vi "Unflatten Waveform Summary JSON.vi"(8 "error in":errorcluster, 11 "Measurement Configuration In":T1={"TDMS File Location"="", "Run Action"="Create/Replace Wfm Group", "Wfm Group Name"="Wfm1", "Channel Names"=[], "Waveforms Summary JSON"=[]}) -> (0 "error out":errorcluster, 2 "Waveforms":waveform(dbl)[](array[waveform]), 3 "Measurement Configuration Out":T1)   [LabVIEW 2025, in "TDMS Waveform Creator.lvclass"]
uses:
  TDMS Waveform Creator.lvclass
  TDMS Waveform Creator.lvclass/TDMS Waveform Creator.ctl
  TDMS Waveform Creator UI/TDMS Waveform Creator UI.lvlib
  Measurement Configuration.ctl
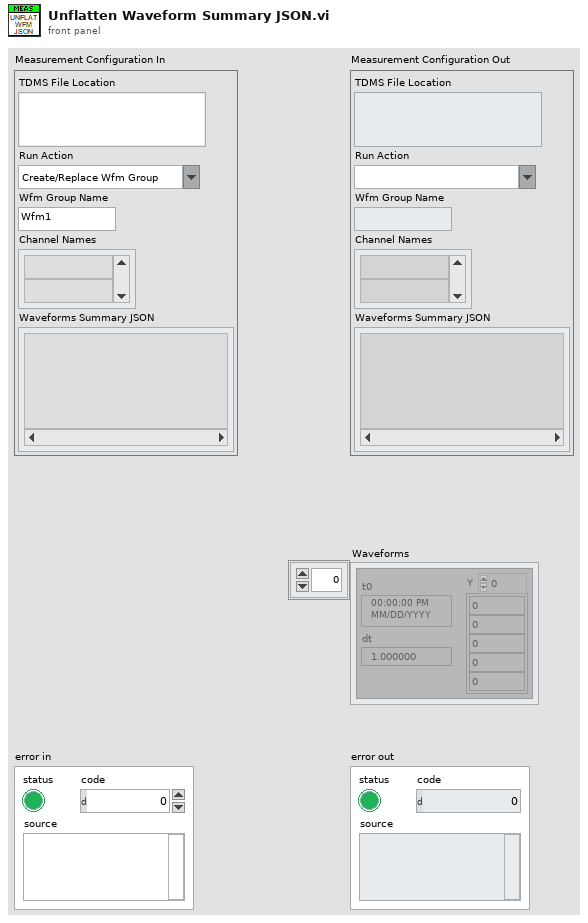
[diagram p1: front panel]
types:
  T1 = typedef "TDMS Waveform Creator.lvclass/Measurement Configuration.ctl" = cluster{"TDMS File Location":string, "Run Action":string, "Wfm Group Name":string, "Channel Names":string[], "Waveforms Summary JSON":string[]}
  T2 = cluster{"Trim and Resample Settings":cluster{"Duration":dbl, "Sample Rate":dbl}, "Wfms Json":string[]}
  T3 = cluster{"File Path":string, "Sample Rate (Hz)":dbl, "Read From":i32, "Pre Delay (s)":dbl, "Post Delay (s)":dbl, "Scale":dbl}
  T4 = cluster{"Waveform Type":i32, "Sample Rate (Hz)":dbl, "Frequency (Hz)":dbl, "Amplitude":dbl, "Number of Cycles":u32, "Ramp Start":dbl, "Ramp Stop":dbl, "Length (s)":dbl, "DC Value":dbl, "Duration (s)":dbl, "Pre Delay (s)":dbl, "Post Delay (s)":dbl}
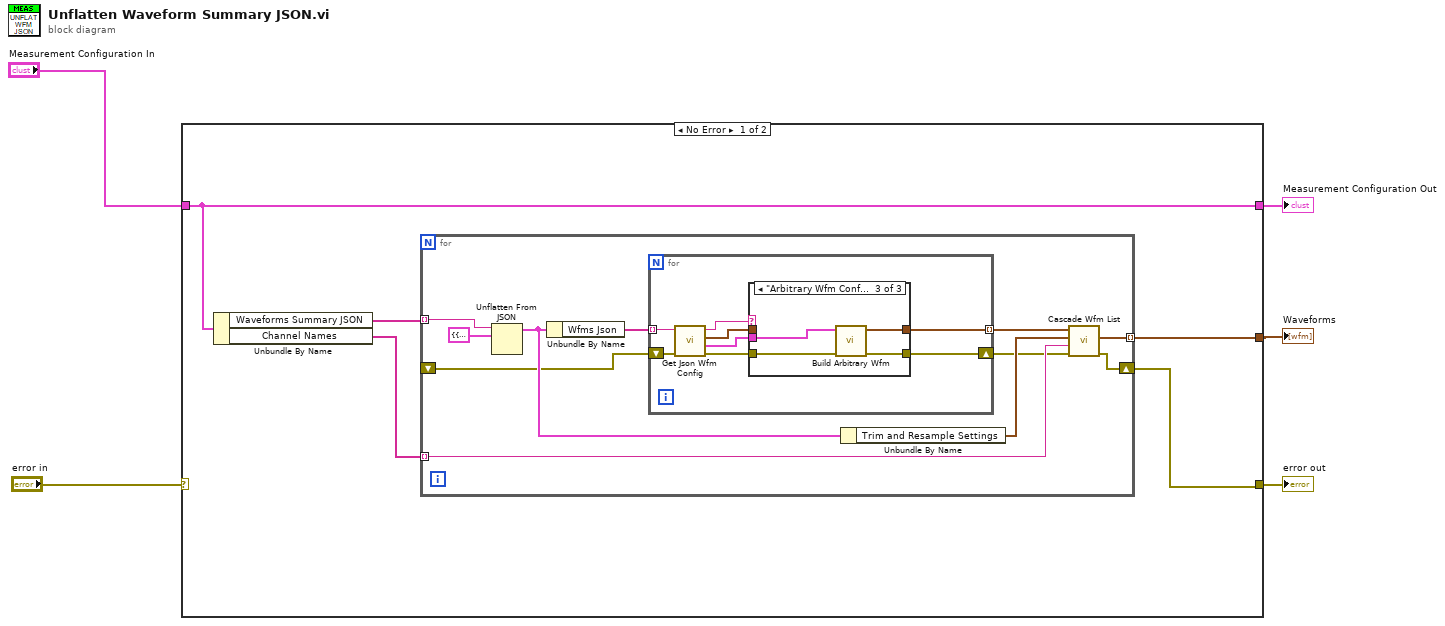
[diagram p0: block diagram]
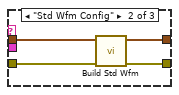
[diagram p3: hidden frame]
diagram:
  n1 = case shown="No Error" "error in" {
    selector: "error in" -> [_ w40]
    tunnel: [w10 w40] -> w4
    tunnel: "Measurement Configuration In" -> [w6 w39]
    tunnel: [w9 _] -> w1
    tunnel: [w6 w39] -> w2
    frame No Error {
      n2 = Unbundle By Name(w6) -> ("Waveforms Summary JSON"=w8:string[], "Channel Names"=w7:string[])
      n3 = for {
        tunnel: w8 -> [w20] mode=indexing
        tunnel: w7 -> [w15] mode=indexing
        tunnel: [w13] -> w9 mode=indexing
        shift-right: [w11] -> w10
        shift-left: _ -> [w12]
        n4 = Unflatten From JSON(JSON string=w20, type and defaults=T2 {"Trim and Resample Settings"={"Duration"=0.0, "Sample Rate"=0.0}, "Wfms Json"=[]} ("Wfm Summary")) -> (value=w17:T2)  [unwired: 5 in, 1 out]
        n5 = Unbundle By Name(w17) -> ("Wfms Json"=w19:string[])
        n6 = for {
          tunnel: w19 -> [w29] mode=indexing
          shift-right: [w24] -> w14
          shift-left: w12 -> [w23]
          tunnel: [w22] -> w18 mode=indexing
          n7 = call "Get Json Wfm Config.vi"("error in"=w23, "Json String"=w29) -> ("error out"=w26:errorcluster, "Arbitrary Wfm Config"=w25:T3, "Std Wfm Config"=w27:T4, "Type"=w28:string)  [unwired: 6 in]
          n8 = case shown="\"Arbitrary Wfm Config\"" w28 {
            tunnel: w27 -> [_ w31 _]
            tunnel: w26 -> [w30 w34 w38]
            tunnel: w25 -> [_ _ w37]
            tunnel: [_ w32 w36] -> w22
            tunnel: [w30 w33 w35] -> w24
            frame Default {
            }
            frame "Std Wfm Config" {
              n9 = call "Build Std Wfm.vi"("error in"=w34, "Standard Wfm Config"=w31) -> ("error out"=w33:errorcluster, "Waveform"=w32:waveform(dbl))  [unwired: 6 in, 2 out]
            }
            frame "Arbitrary Wfm Config" {
              n10 = call "Build Arbitrary Wfm.vi"("error in"=w38, "Arbitrary Wfm Config"=w37) -> ("error out"=w35:errorcluster, "Waveform"=w36:waveform(dbl))  [unwired: 6 in, 2 out]
            }
          }
        }
        n11 = Unbundle By Name(w17) -> ("Trim and Resample Settings"=w16:cluster{"Duration":dbl, "Sample Rate":dbl})
        n12 = call "Cascade Wfm List.vi"("error in (no error)"=w14, "Channel Name"=w15, "Trim and Resample Settings"=w16, "Canvas Wfm Array In"=w18) -> ("error out"=w11:errorcluster, "Final Flatten Wfm Channel"=w13:waveform(dbl))  [unwired: 5 in, 1 out]
      }
    }
    frame Error {
    }
  }
  "error out" <- w4
  "Measurement Configuration Out" <- w2
  "Waveforms" <- w1
